vi "Initialize Instrument.vi"(8 "error in (no error)":errorcluster, 10 "Instr Resource Str":string, 11 "Ag Sig Gen.lvclass in":refnum<class "Ag Sig Gen.lvclass">) -> (0 "error out":errorcluster, 3 "Ag Sig Gen.lvclass out":refnum<class "Ag Sig Gen.lvclass">)   [LabVIEW 2010, in "Ag Sig Gen.lvclass"]
uses:
  Ag Sig Gen.lvclass
  Ag Sig Gen.lvclass/Ag Sig Gen.ctl
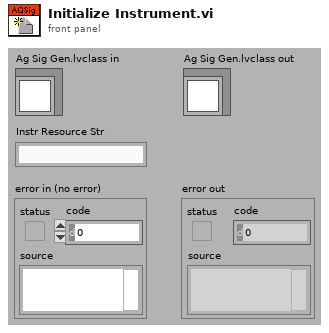
[diagram p1: front panel]
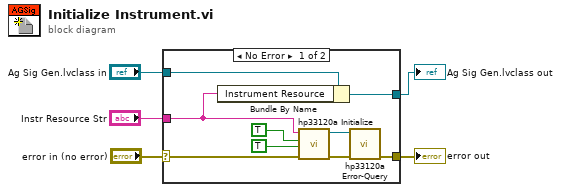
[diagram p0: block diagram]
diagram:
  n1 = case shown="No Error" "error in (no error)" {
    selector: "error in (no error)" -> [w12 w16]
    tunnel: [w13 w16] -> w5
    tunnel: "Instr Resource Str" -> [w6 _]
    tunnel: "Ag Sig Gen.lvclass in" -> [w8 w15]
    tunnel: [w7 w15] -> w2
    frame No Error {
      n2 = Bundle By Name(cluster=w8, "Instrument Resource"=w6) -> (w7:refnum<class "Ag Sig Gen.lvclass">)
      n3 = call <instrlib>:"hp33120a Initialize.vi"("error in (no error)"=w12, "reset device (True)"=TRUE ("Reset? (T: Yes)"), "id query (True)"=TRUE ("ID Query? (T: Yes)"), "resource name"=w6) -> ("error out"=w10:errorcluster, "Instrument Handle out"=w11:refnum<k15>)  [unwired: 6 out]
      n4 = call <instrlib>:"hp33120a Error-Query.vi"("error in (no error)"=w10, "instrument handle"=w11) -> ("error out"=w13:errorcluster)  [unwired: 9 out]
    }
    frame Error {
    }
  }
  "error out" <- w5
  "Ag Sig Gen.lvclass out" <- w2
